vi "writeExcel.vi"(8 "template (empty)":path caption="模板（空）", 9 "枚举":enum16{"", "写", "读"}(ring), 10 "formula":string, 11 "start (0, 0)":cluster{"row":i32, "column":i32}) -> (2 "data":string)   [LabVIEW 2018]
uses:
  <vilib>/Utility/NIReport.llb/Report Type.ctl
  <vilib>/addons/_office/excel.llb/Excel Get Data (str).vi
  <vilib>/Utility/NIReport.llb/NI_report.lvclass
  <vilib>/Utility/NIReport.llb/NI_ReportGenerationCore.lvlib
  <vilib>/Utility/NIReport.llb/Excel/NI_Excel.lvclass
  <vilib>/addons/_office/NI_ReportGenerationToolkit.lvlib
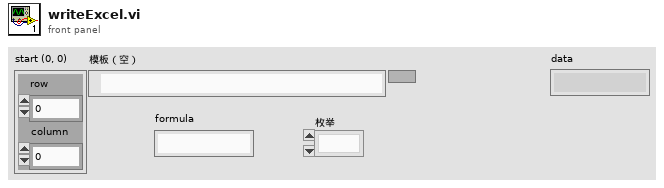
[diagram p1: front panel]
types:
  T1 = typedef "NI_ReportGenerationCore.lvlib/Report Type.ctl" = enum16{"HTML", "Word", "Excel"}
  T2 = enum16{"maximized", "minimized", "normal", "no change"}
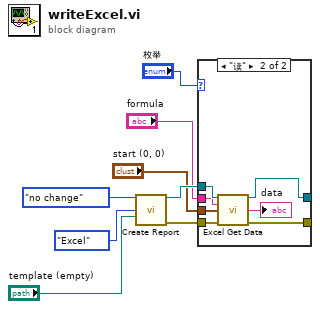
[diagram p0: block diagram]
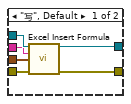
[diagram p2: hidden frame]
diagram:
  n1 = call <vilib>:"Create Report.vi"("window state (normal)"=T2."no change", "report type"=Report_Type."Excel", "template (empty)"="template (empty)") -> ("report out"=w6:refnum<class "NI_report.lvclass">, "error out"=w5:errorcluster)  [unwired: 11 in]
  n2 = case shown="\"读\"" "枚举" {
    tunnel: [w14 w18] -> _
    tunnel: [w13 w20] -> _
    tunnel: w6 -> [w12 w21]
    tunnel: w5 -> [w11 w19]
    tunnel: "start (0, 0)" -> [w10 w17]
    tunnel: "formula" -> [w9 w16]
    frame "写", Default {
      n3 = call <vilib>:"Excel Insert Formula.vi"("report in"=w12, "formula"=w9, "start (0, 0)"=w10, "error in (no error)"=w11) -> ("report out"=w13:refnum<class "NI_report.lvclass">, "error out"=w14:errorcluster)  [unwired: 10 in]
    }
    frame "读" {
      n4 = call-poly <vilib>:"Excel Get Data.vi"("report in"=w21, "data type"=w16, "start (0, 0)"=w17, "error in (no error)"=w19) -> ("report out"=w20:refnum<class "NI_report.lvclass">, "data"=→"data":string, "error out"=w18:errorcluster)  [unwired: 9 in]
    }
  }
